vi "Set Receiver.vi"(0 "TSM Context In":T2, 1 "RFPM Parameters":T1={"Disconnect SG PM Path?"=FALSE, "SG PM Path"=3, "SG Amplitude Settling (dB)"=0.0, "SG Path Optimization Method"=0, "SA PM Path"=3, "SA PM Coupling Path"=3, "SA Amplitude Settling (dB)"=0.0, "SA Path Optimization Method"=0} {"SA Path Optimization Method" items=["Normal", "Optimize for Dynamic Range"]; "SA PM Coupling Path" items=["Auto"=3, "LNA"=2, "Direct"=0, "Coupled"=1]; "SA PM Path" items=["Auto"=3, "Loop"=2, "Gain"=1, "Direct"=0]; "SG Path Optimization Method" items=["Normal", "Optimize for Dynamic Range"]; "SG PM Path" items=["Auto"=3, "Loop"=2, "Gain"=1, "Direct"=0]}, 2 "Enable S2P De-embedding?":bool, 5 "Pin":tag, 11 "error in":errorcluster, 12 "PAPR":dbl) -> (4 "TSM Context Out":T2, 6 "RFPM Handle":refnum<k15>, 15 "error out":errorcluster)   [LabVIEW 2023, in "RFFixtureCharact.RFPM.lvlib" / "RF Subsystem Session Provider.lvclass"]
uses:
  RF Subsystem Session Provider.lvclass
  <vilib>/NI_TestStand_SemiconductorModule/NI_TestStand_Semiconductor_Module.lvlibp/PinMap/General/SemiconductorModuleContext.ctl
  Controls/RFPM Parameters.ctl
  <vilib>/NI_TestStand_SemiconductorModule/NI_TestStand_Semiconductor_Module.lvlibp/PinMap/RF/RFPM/PinToNIRFPMSessionsWithPaths.vi
  <vilib>/NI_TestStand_SemiconductorModule/NI_TestStand_Semiconductor_Module.lvlibp
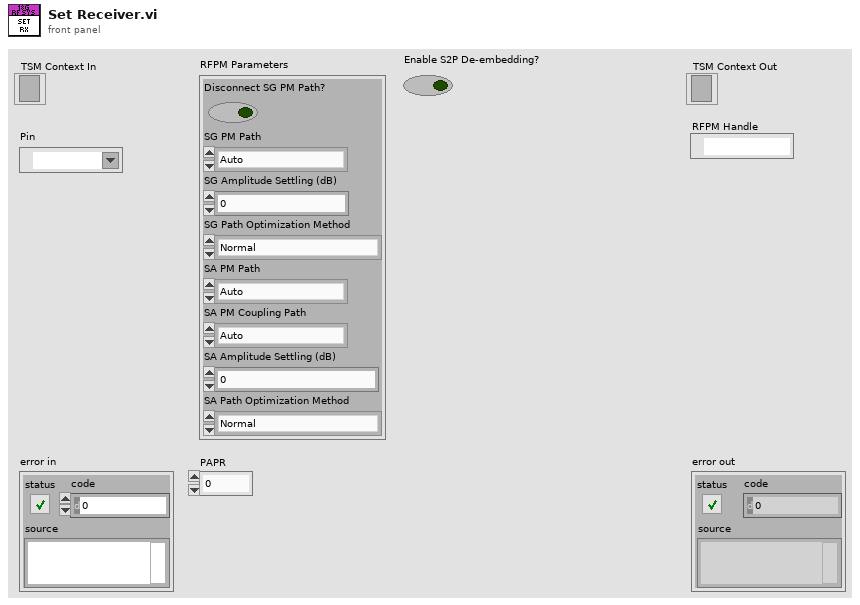
[diagram p1: front panel]
types:
  T1 = typedef "RFFixtureCharact.RFPM.lvlib/RF Subsystem Session Provider.lvclass/RFPM Parameters.ctl" = cluster{"Disconnect SG PM Path?":bool, "SG PM Path":u32, "SG Amplitude Settling (dB)":dbl, "SG Path Optimization Method":i32, "SA PM Path":u32, "SA PM Coupling Path":u32, "SA Amplitude Settling (dB)":dbl, "SA Path Optimization Method":i32}
  T2 = typedef "NI_TestStand_Semiconductor_Module.lvlibp/SemiconductorModuleContext.ctl" = refnum<k7>
  T3 = typedef "NI_TestStand_Semiconductor_Module.lvlibp/DeembeddingFile.ctl" = cluster{" Path":path, "Orientation":i32}
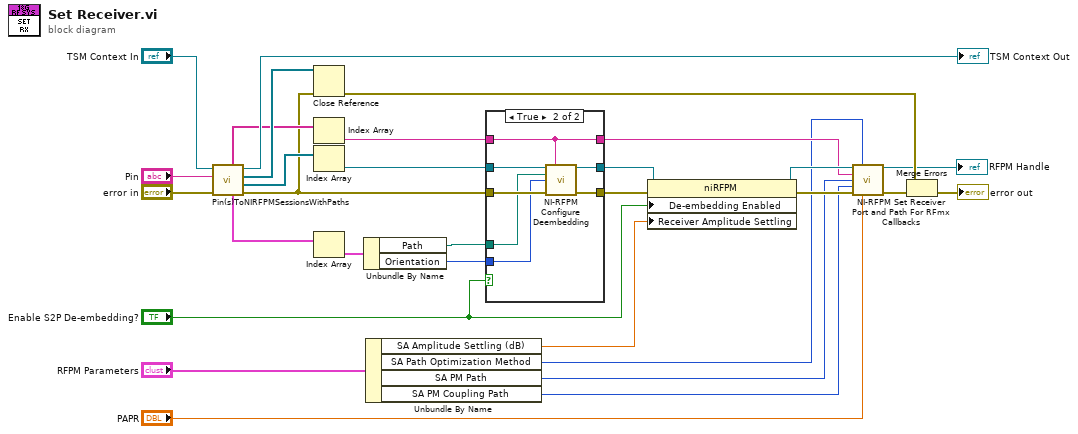
[diagram p0: block diagram]
diagram:
  n1 = call-poly <vilib>:"Pin(s)ToNIRFPMSessionsWithPaths.vi"("error in (no error)"="error in", "Pin"="Pin", "Semiconductor Module Context"="TSM Context In") -> ("error out"=w12:errorcluster, "Instrument Sessions"=w24:refnum<k15>[], "Semiconductor Module Contexts"=w26:T2[], "Semiconductor Module Context out"=→"TSM Context Out":T2, "De-embedding Files"=w23:T3[], "Ports List"=w25:string[])  [unwired: 3 in]
  n2 = Close Reference(reference=w26, error in (no error)=w12) -> (error out=w8:errorcluster)
  n3 = Index Array(array=w25) -> (element=w19:string)  [unwired: 1 in]
  n4 = Index Array(array=w24) -> (element=w21:refnum<k15>)  [unwired: 1 in]
  n5 = Index Array(array=w23) -> (element=w22:T3)  [unwired: 1 in]
  n6 = Unbundle By Name(w22) -> ("Path"=w2:path, "Orientation"=w20:i32)
  n7 = Unbundle By Name("RFPM Parameters") -> ("SA Amplitude Settling (dB)"=w4:dbl, "SA Path Optimization Method"=w7:i32, "SA PM Path"=w14:u32, "SA PM Coupling Path"=w5:u32)
  n8 = case shown="True" "Enable S2P De-embedding?" {
    tunnel: w12 -> [w32 w39]
    tunnel: w21 -> [w33 w40]
    tunnel: w20 -> [_ w38]
    tunnel: w19 -> [w31 w35]
    tunnel: [w32 w37] -> w17
    tunnel: [w33 w36] -> w18
    tunnel: [w31 w35] -> w11
    tunnel: w2 -> [_ w34]
    frame False {
    }
    frame True {
      n9 = call <instrlib>:"NI-RFPM Configure Deembedding.vi"("instrument handle"=w40, "port"=w35, "Deembedding S2P File Path"=w34, "Deembedding Orientation"=w38, "error in (no error)"=w39) -> ("instrument handle out"=w36:refnum<k15>, "error out"=w37:errorcluster)  [unwired: 9 in]
    }
  }
  n10 = property class="niRFPM"(reference=w18, error in=w17, "De-embedding Enabled"="Enable S2P De-embedding?", "Receiver Amplitude Settling"=w4) -> (reference out=w15:refnum<k15>, error out=w16:errorcluster)
  n11 = call <instrlib>:"NI-RFPM Set Receiver Port and Path For RFmx Callbacks.vi"("instrument handle"=w15, "Optimization Method"=w7, "Port"=w11, "Receiver Path"=w14, "Receiver Coupling Path"=w5, "error in"=w16, "PAPR"="PAPR") -> ("instrument handle out"=→"RFPM Handle":refnum<k15>, "error out"=w6:errorcluster)  [unwired: 7 in]
  n12 = Merge Errors(w8, w6) -> (→"error out":errorcluster)
